vi "Get_Psi_U_coeffs.vi"(1 "file path (dialog if empty)":path) -> (0 "Coeffs to append":dbl[](array[numeric]))   [LabVIEW 2010]
uses:
  <vilib>/Utility/file.llb/Read From Spreadsheet File (string).vi
panel:
  out "all rows":string[][](array[string])
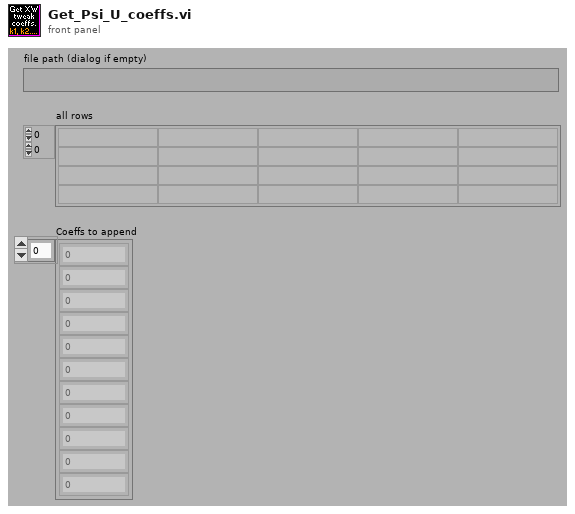
[diagram p1: front panel]
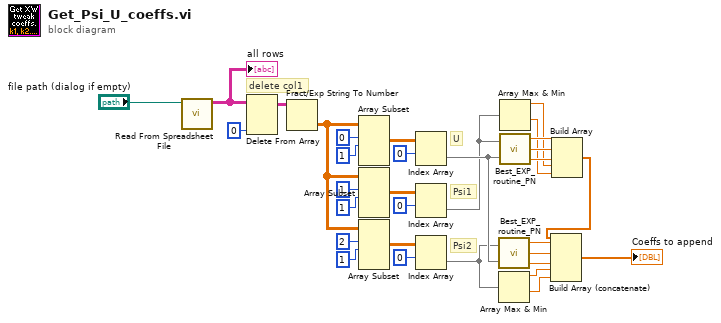
[diagram p0: block diagram]
diagram:
  # "delete col1"
  # "Psi2"
  # "Psi1"
  # "U"
  n1 = call-poly <vilib>:"Read From Spreadsheet File.vi"("file path (dialog if empty)"="file path (dialog if empty)") -> ("all rows"=w31:string[][])  [unwired: 3 in, 7 out]
  "all rows" <- w31
  n2 = Delete From Array(array=w31, index (col)=0 ("disabled index (col)")) -> (array with subset deleted=w25:string[][])  [unwired: 2 in, 1 out]
  n3 = Fract/Exp String To Number(string=w25) -> (number=w16:dbl[][])  [unwired: 4 out]
  n4 = Array Subset(array=w16, index (row)=0 ("index"), length (row)=1 ("length")) -> (w27:dbl[][])  [unwired: 2 in]
  n5 = Array Subset(array=w16, index (row)=1 ("index"), length (row)=1 ("length")) -> (w23:dbl[][])  [unwired: 2 in]
  n6 = Array Subset(array=w16, index (row)=2 ("index"), length (row)=1 ("length")) -> (w18:dbl[][])  [unwired: 2 in]
  n7 = Index Array(array=w27, index (row)=0) -> (element=w15:dbl[])  [unwired: 1 in]
  n8 = Index Array(array=w23, index (row)=0) -> (element=w14:dbl[])  [unwired: 1 in]
  n9 = Index Array(array=w18, index (row)=0) -> (element=w13:dbl[])  [unwired: 1 in]
  n10 = call "Best_EXP_routine_PN.vi"("Psi"=w13, "U"=w15) -> ("k1"=w7:dbl, "k2"=w6:dbl, "k3"=w5:dbl)
  n11 = Array Max & Min(array=w13) -> (max value=w4:dbl, min value=w3:dbl)  [unwired: 2 out]
  n12 = Array Max & Min(array=w14) -> (max value=w9:dbl, min value=w8:dbl)  [unwired: 2 out]
  n13 = call "Best_EXP_routine_PN.vi"("Psi"=w14, "U"=w15) -> ("k1"=w12:dbl, "k2"=w11:dbl, "k3"=w10:dbl)
  n14 = Build Array(w12, w11, w10, w9, w8) -> (w2:dbl[])
  n15 = Build Array (concatenate)(w2, w7, w6, w5, w4, w3) -> (→"Coeffs to append":dbl[])
